vi "USB_DAQ__DS3231_RTC_Test_WRITE_Date_Time.vi"() -> ()   [LabVIEW 2022 SP3]
doc: "Petrus Prins \n26 July 2026"
panel:
  out "Page.ACK0":bool
  in  "Page.Address0":u8 format="%02x"
  out "Data.ACK":bool
  in  "Data.Byte":u8=65 format="%02x"
  out "RunTime.ms":u32
  in  "Page.Address1":u8 format="%02x"
  out "Page.ACK1":bool
  out "Addr.ACK":bool
  in  "24C32.Address":u8=87 format="%02x"
  in  "Write":bool
  # "EEPROM 24C32 WRITE"
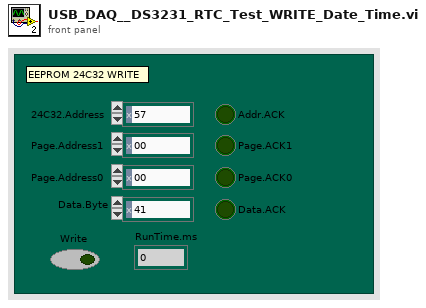
[diagram p1: front panel]
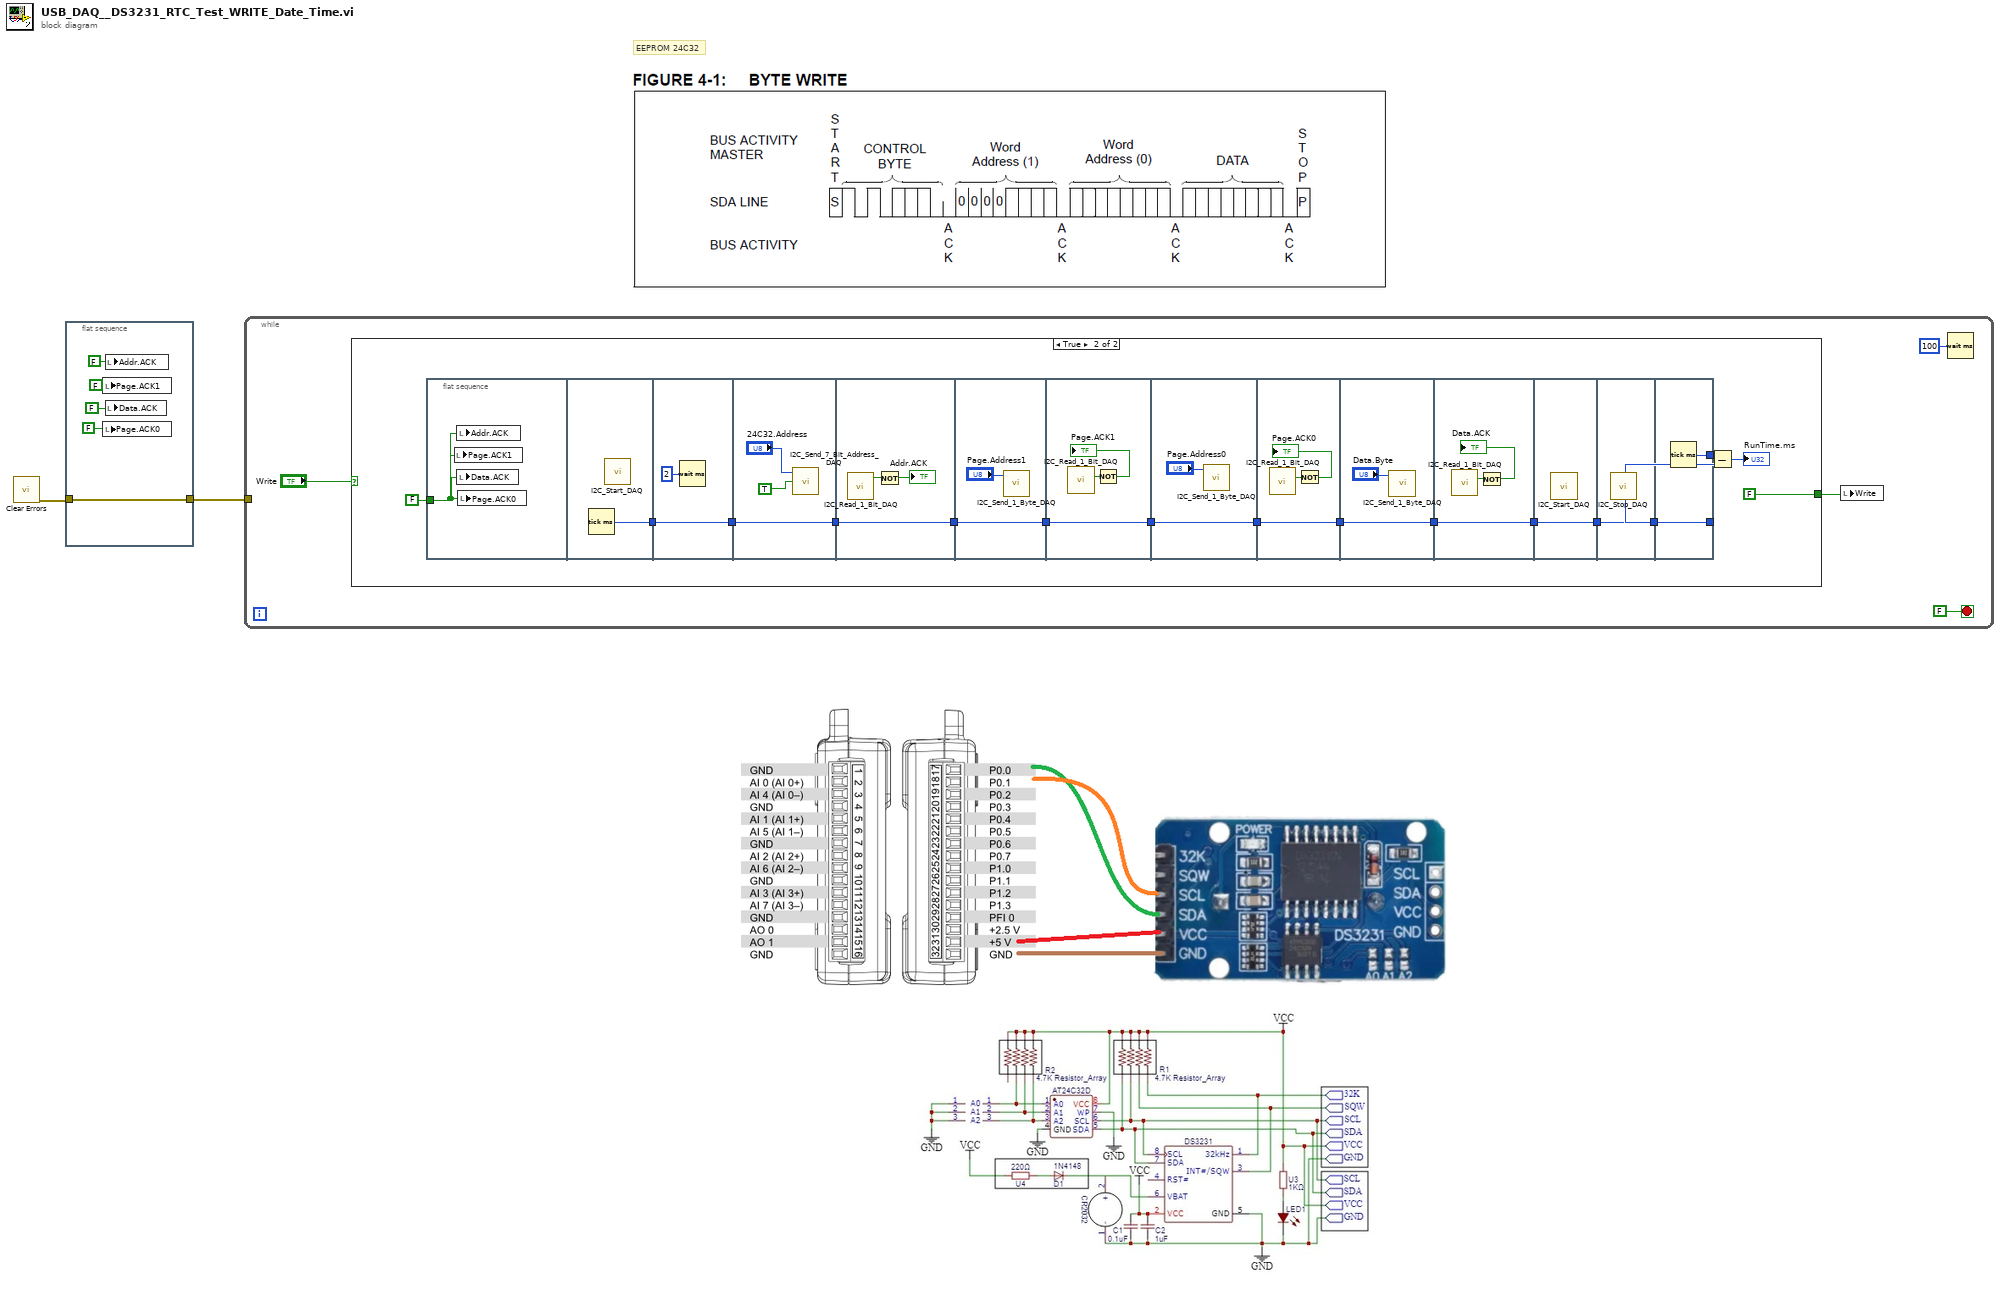
[diagram p0: block diagram]
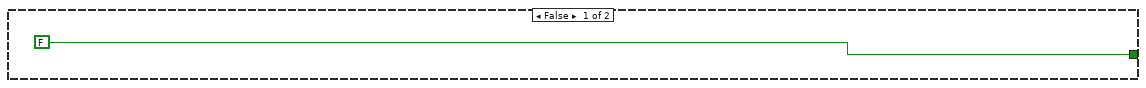
[diagram p2: hidden frame]
diagram:
  # "EEPROM 24C32"
  n1 = call <vilib>:"Clear Errors.vi"() -> ("error out"=w1:errorcluster)  [unwired: 6 in, 1 out]
  n2 = flat-sequence {
    tunnel: w1 -> [w7]
    tunnel: [w7] -> w2
    frame #0 {
      n3 = local write "Page.ACK1"(FALSE ("TX.ACK")) -> ()
      n4 = local write "Page.ACK0"(FALSE ("Page.ACK0")) -> ()
      n5 = local write "Addr.ACK"(FALSE ("ACK_OK")) -> ()
      n6 = local write "Data.ACK"(FALSE ("Data.ACK")) -> ()
    }
  }
  n7 = while {
    tunnel: w2 -> [_]
    stop <- FALSE stop-if-true
    n8 = case shown="True" "Write" {
      tunnel: [FALSE ("Test") FALSE ("Test")] -> w8
      frame False {
      }
      frame True {
        n9 = flat-sequence {
          tunnel: FALSE ("Data.ACK") -> [w30]
          tunnel: [w31] -> w20
          tunnel: [w32] -> w21
          tunnel: w20 -> [w32]
          tunnel: [w34] -> w22
          tunnel: w21 -> [w34]
          tunnel: [w37] -> w23
          tunnel: w22 -> [w37]
          tunnel: [w40] -> w24
          tunnel: w23 -> [w40]
          tunnel: [w42] -> w16
          tunnel: w24 -> [w42]
          tunnel: w16 -> [w46]
          tunnel: [w46] -> w15
          tunnel: w15 -> [w49]
          tunnel: [w49] -> w14
          tunnel: [w50] -> w25
          tunnel: w14 -> [w50]
          tunnel: [w52] -> w26
          tunnel: w25 -> [w52]
          tunnel: [w55] -> w27
          tunnel: w26 -> [w55]
          tunnel: [w56] -> w28
          tunnel: w27 -> [w56]
          tunnel: w28 -> [w57]
          tunnel: [w58] -> w18
          tunnel: [w57] -> w17
          frame #0 {
            n10 = local write "Page.ACK1"(w30) -> ()
            n11 = local write "Addr.ACK"(w30) -> ()
            n12 = local write "Data.ACK"(w30) -> ()
            n13 = local write "Page.ACK0"(w30) -> ()
          }
          frame #1 {
            n14 = Tick Count (ms)() -> (millisecond timer value=w31:u32)
            n15 = call "I2C_Start_DAQ.vi"() -> ()  [unwired: 6 in]
          }
          frame #2 {
            n16 = Wait (ms)(milliseconds to wait=u32 2) -> ()  [unwired: 1 out]
          }
          frame #3 {
            n17 = call "I2C_Send_7_Bit_Address_DAQ.vi"("Write or Read?"=TRUE, "Receiver_7_Bit_Address"="24C32.Address") -> ()  [unwired: 1 in]
          }
          frame #4 {
            n18 = call "I2C_Read_1_Bit_DAQ.vi"() -> ("RX_Bit_Out"=w39:bool)  [unwired: 2 in]
            n19 = Not(x=w39) -> (.not. x?=→"Addr.ACK":bool)
          }
          frame #5 {
            n20 = call "I2C_Send_1_Byte_DAQ.vi"("Byte_To_Send"="Page.Address1") -> ()  [unwired: 2 in]
          }
          frame #6 {
            n21 = call "I2C_Read_1_Bit_DAQ.vi"() -> ("RX_Bit_Out"=w44:bool)  [unwired: 2 in]
            n22 = Not(x=w44) -> (.not. x?=→"Page.ACK1":bool)
          }
          frame #7 {
            n23 = call "I2C_Send_1_Byte_DAQ.vi"("Byte_To_Send"="Page.Address0") -> ()  [unwired: 2 in]
          }
          frame #8 {
            n24 = call "I2C_Read_1_Bit_DAQ.vi"() -> ("RX_Bit_Out"=w48:bool)  [unwired: 2 in]
            n25 = Not(x=w48) -> (.not. x?=→"Page.ACK0":bool)
          }
          frame #9 {
            n26 = call "I2C_Send_1_Byte_DAQ.vi"("Byte_To_Send"="Data.Byte") -> ()  [unwired: 2 in]
          }
          frame #10 {
            n27 = call "I2C_Read_1_Bit_DAQ.vi"() -> ("RX_Bit_Out"=w53:bool)  [unwired: 2 in]
            n28 = Not(x=w53) -> (.not. x?=→"Data.ACK":bool)
          }
          frame #11 {
            n29 = call "I2C_Start_DAQ.vi"() -> ()  [unwired: 6 in]
          }
          frame #12 {
            n30 = call "I2C_Stop_DAQ.vi"() -> ()  [unwired: 6 in]
          }
          frame #13 {
            n31 = Tick Count (ms)() -> (millisecond timer value=w58:u32)
          }
        }
        n32 = Subtract(x=w18, y=w17) -> (x-y=→"RunTime.ms":u32)
      }
    }
    n33 = local write "Write"(w8) -> ()
    n34 = Wait (ms)(milliseconds to wait=u32 100) -> ()  [unwired: 1 out]
  }
